vi "Inline Read.vi"(1 "RT Data in":T1 {"Device Channels"."Status"."BD Refs"."Data Reference" format="%.0x"; "Device Channels"."Command"."BD Refs"."Data Reference" format="%.0x"; "Local Chassis"."FPGA"."VS ref" format="%.0x"; "Local Chassis"."RSI Modules"."VS ref" format="%.0x"; "Local Chassis"."VS ref" format="%.0x"; "Device ref" format="%.0x"; "EtherCAT Masters"."DS402 Drive ECAT Slaves"."VS ref" format="%.0x"; "EtherCAT Masters"."REM IO ECAT Slaves"."VS ref" format="%.0x"; "EtherCAT Masters"."Generic EtherCAT Slaves"."VS ref" format="%.0x"; "EtherCAT Masters"."VS ref" format="%.0x"; "EtherCAT Masters"."EtherCAT Slaves"."FPGA"."VS ref" format="%.0x"; "EtherCAT Masters"."EtherCAT Slaves"."RSI Modules"."VS ref" format="%.0x"; "EtherCAT Masters"."EtherCAT Slaves"."VS ref" format="%.0x"}) -> (0 "RT Data out":T1 {"Device Channels"."Status"."BD Refs"."Data Reference" format="%.0x"; "Device Channels"."Command"."BD Refs"."Data Reference" format="%.0x"; "Local Chassis"."FPGA"."VS ref" format="%.0x"; "Local Chassis"."RSI Modules"."VS ref" format="%.0x"; "Local Chassis"."VS ref" format="%.0x"; "Device ref" format="%.0x"; "EtherCAT Masters"."DS402 Drive ECAT Slaves"."VS ref" format="%.0x"; "EtherCAT Masters"."REM IO ECAT Slaves"."VS ref" format="%.0x"; "EtherCAT Masters"."Generic EtherCAT Slaves"."VS ref" format="%.0x"; "EtherCAT Masters"."VS ref" format="%.0x"; "EtherCAT Masters"."EtherCAT Slaves"."FPGA"."VS ref" format="%.0x"; "EtherCAT Masters"."EtherCAT Slaves"."RSI Modules"."VS ref" format="%.0x"; "EtherCAT Masters"."EtherCAT Slaves"."VS ref" format="%.0x"})   [LabVIEW 2016, in "Scan Engine Custom Device.lvlib"]
uses:
  Scan Engine Custom Device.lvlib
  Type Defs/RT Data.ctl
  <vilib>/NI Veristand/Custom Device API/Custom Device Item Ref.ctl
  Type Defs/Device Channels.ctl
  Type Defs/Output Data.ctl
  <vilib>/NI Veristand/Custom Device API/Block Data Reference.ctl
  <vilib>/NI Veristand/Custom Device API/Data Reference.ctl
  Type Defs/Input Data.ctl
  Type Defs/Local Chassis Data.ctl
  Type Defs/RSI Module Data.ctl
  Type Defs/Open Module IOVs.ctl
  Modules.lvlibp/RSI Module/RSI Module.lvclass
  Modules.lvlibp/RSI Module/Module Models.ctl
  Modules.lvlibp/RSI Module/Channel Type.ctl
  Type Defs/Module Config Data.ctl
  Type Defs/Mixed IO.ctl
  Type Defs/FPGA Data.ctl
  Type Defs/UDV Data.ctl
  Type Defs/UDV Data Type.ctl
  Type Defs/FXP Config.ctl
  Type Defs/Mod Size Indexes.ctl
  Type Defs/EtherCAT Master Data.ctl
  Type Defs/EtherCAT Slave Data.ctl
  Type Defs/Generic ECAT Slave RT-Data-Array.ctl
  Type Defs/Generic ECAT Slave Data Cluster.ctl
  Type Defs/Generic ECAT Slave IOV Cluster.ctl
  Type Defs/REM IO ECAT Slave RT-Data-Array.ctl
  Type Defs/REM IO ECAT Slave Data Cluster.ctl
  Type Defs/REM IO ECAT Slave IOV Cluster.ctl
  Type Defs/DS402 Drive ECAT Slave RT-Data-Array.ctl
  Type Defs/DS402 Drive ECAT Slave Data Cluster.ctl
  Type Defs/DS402 Drive ECAT Slave IOV Cluster.ctl
  Type Defs/DS402 Drive ECAT Slave Action IOV Cluster.ctl
  Type Defs/Async Data.ctl
  Type Defs/Async Status.ctl
  Type Defs/Async State.ctl
  Type Defs/Async Command.ctl
  Type Defs/ECAT Reconfig Data.ctl
  Type Defs/ECAT Reconfig Status.ctl
  Type Defs/ECAT Reconfig State.ctl
  Type Defs/RW Case.ctl
  RW All Local.vi
  RW All ECAT.vi
  Check Command Channels.vi
  Read Async FIFOs.vi
  Update Status Channels.vi
  Module Reconfig/Check ECAT Reconfig.vi
  Write Async FIFOs.vi
  RW Local Chassis.vi
  RW Slave.vi
  RW Generic Slaves.vi
  RW Rem IO Slaves.vi
  RW DS402 Drive Slaves.vi
  <vilib>/NI Veristand/Custom Device API/NI VeriStand - Get Channel Values by Block Data Reference.vi
  <vilib>/NI Veristand/Custom Device API/NI VeriStand - Set Channel Values by Block Data Reference.vi
  RW UDVs.vi
  RW Mods.vi
  Read ECAT VARs.vi
  Write ECAT VARs.vi
  Read REM IO VARs.vi
  Write REM IO VARs.vi
  Read DS402 Drive VARs.vi
  Write DS402 Drive VARs.vi
  Read UDVs.vi
  Write UDVs.vi
  Read All Input Module Sizes.vi
  Read All Mixed Module Sizes.vi
  Write Module.vi
  Check Module Config.vi
  Scanned Read - UDV.vi
  Scanned Write - UDV.vi
  Read Input Modules at Indexes.vi
  Read Mixed Modules at Indexes.vi
  Scanned Write - Module.vi
  Read Input Module.vi
  Read Mixed Module.vi
  Scanned Read - Input Module.vi
  Scanned Read - Mixed Module.vi
  <vilib>/NI Veristand/Custom Device API/Global Data Refs.vi
  Module Reconfig/Set ECAT Reconfig Status.vi
  <vilib>/NI/syslog/Syslog Device Send.vi
  Launch Local Reconfig.vi
  DS402 StateMachine/Process DS402 SM.vi
  Async/Set Async Status.vi
  Launch ECAT Reconfig.vi
  Globals/Error Strings.vi
  Module Reconfig/Get ECAT Reconfig Status.vi
  Get Scan Mode.vi
  <vilib>/NI Veristand/Custom Device API/Custom Device API.lvlib
types:
  T1 = typedef "Scan Engine Custom Device.lvlib/RT Data.ctl" = cluster{"Device ref":T2, "Scan Period (uSec)":u32, "Device Channels":T3, "Local Chassis":T8[], "EtherCAT Masters":T20[], "Async":T32, "ECAT Reconfig":T33, "Device Error":errorcluster, "DeviceName":string, "PCLSync?":bool}
  T2 = typedef "Custom Device API.lvlib/Custom Device Item Ref.ctl" = u64
  T3 = typedef "Scan Engine Custom Device.lvlib/Device Channels.ctl" = cluster{"Status":T4, "Command":T7}
  T4 = typedef "Scan Engine Custom Device.lvlib/Output Data.ctl" = cluster{"BD Refs":T5[], "Length":i32, "FIFO Index":i32, "Data":dbl[]}
  T5 = typedef "Custom Device API.lvlib/Block Data Reference.ctl" = cluster{"Data Reference":T6, "Offset":u64, "Length":u64}
  T6 = typedef "Custom Device API.lvlib/Data Reference.ctl" = i32
  T7 = typedef "Scan Engine Custom Device.lvlib/Input Data.ctl" = cluster{"BD Refs":T5[], "Data":dbl[], "Length":i32, "FIFO Index":i32}
  T8 = typedef "Scan Engine Custom Device.lvlib/Local Chassis Data.ctl" = cluster{"VS ref":T2, "RSI Modules":T9[], "FPGA":T15[], "Input Mod Size Idxs":T19, "Output Modules":i32[], "MixedIO Mod Size Idxs":T19}
  T9 = typedef "Scan Engine Custom Device.lvlib/RSI Module Data.ctl" = cluster{"VS ref":T2, "IOV ref":refnum<k21>, "Open Mod refs":T10, "Module DVR":refnum<data-value>, "Slot":u32, "Model":T11, "Channel Type":T12, "EtherCAT?":bool, "CDInput Data":T7, "CDOutput Data":T4, "Module Config Data":T13, "Mixed IO":T14}
  T10 = typedef "Scan Engine Custom Device.lvlib/Open Module IOVs.ctl" = cluster{"Analog Read":refnum<k21>, "Digital Read":refnum<k21>, "Analog Write":refnum<k21>, "Digital Write":refnum<k21>}
  T11 = typedef "Modules.lvlibp/RSI Module.lvclass/Module Models.ctl" = enum16{"Empty", "NI 9201", "NI 9203", "NI 9205", "NI 9206", "NI 9207", "NI 9208", "NI 9211", "NI 9212", "NI 9213", "NI 9214", "NI 9215", "NI 9217", "NI 9219", "NI 9220", "NI 9221", "NI 9222", "NI 9223", "NI 9225", "NI 9227", "NI 9229", "NI 9233", "NI 9234", "NI 9235", "NI 9236", "NI 9237", "NI 9239", "NI 9242", "NI 9244", "NI 9263", "NI 9264", "NI 9265", "NI 9269", "NI 9375", "NI 9401", "NI 9402", "NI 9403", "NI 9411", "NI 9421", "NI 9422", "NI 9423", "NI 9425", "NI 9426", "NI 9435", "NI 9437", "NI 9472", "NI 9474", "NI 9475", "NI 9476", "NI 9477", "NI 9478", "NI 9481", "NI 9482", "NI 9485"}
  T12 = typedef "Modules.lvlibp/RSI Module.lvclass/Channel Type.ctl" = enum16{"Analog", "Digital"}
  T13 = typedef "Scan Engine Custom Device.lvlib/Module Config Data.ctl" = cluster{"Configurable?":bool, "Config Block Data Refs":T5[], "Config Data DVR":refnum<data-value>, "Previous Values":dbl[], "Local Reconfig VI Ref":refnum<vi>}
  T14 = typedef "Scan Engine Custom Device.lvlib/Mixed IO.ctl" = cluster{"Input Channel Indices":i32[], "Input Buffer":dbl[]}
  T15 = typedef "Scan Engine Custom Device.lvlib/FPGA Data.ctl" = cluster{"VS ref":T2, "IOV ref":refnum<k21>, "FPGA Target":enum16{"Local", "EtherCAT"}, "Product Code":u32, "Bitfile Signature":string, "Bitfile Path (RT)":path, "FPGA Session":u32, "Input Data":T7, "Output Data":T4, "UDVs":cluster{"From FPGA":T16[], "To FPGA":T16[]}}
  T16 = typedef "Scan Engine Custom Device.lvlib/UDV Data.ctl" = cluster{"VS ref":T2, "IOV Ref":refnum<k21>, "Name":string, "UDV Data Type":T17, "Supported Type?":bool, "FXP Config":T18, "FXP VI Ref":refnum<vi>}
  T17 = typedef "Scan Engine Custom Device.lvlib/UDV Data Type.ctl" = enum16{"Boolean", "Fixed Point", "Int8", "Int16", "Int32", "Int64", "U32 Bit Field", "UInt8", "UInt16", "UInt32", "UInt64", "Other"}
  T18 = typedef "Scan Engine Custom Device.lvlib/FXP Config.ctl" = cluster{"signed":bool, "size":u32, "integersize":i32}
  T19 = typedef "Scan Engine Custom Device.lvlib/Mod Size Indexes.ctl" = cluster{"4":i32[], "8":i32[], "16":i32[], "32":i32[], "other":i32[]}
  T20 = typedef "Scan Engine Custom Device.lvlib/EtherCAT Master Data.ctl" = cluster{"VS ref":T2, "IOV ref":refnum<k21>, "Master ID":u32, "Cyclic Data Bandwidth":u32, "EtherCAT Slaves":T21[], "Generic EtherCAT Slaves":T22, "REM IO ECAT Slaves":T25, "DS402 Drive ECAT Slaves":T28}
  T21 = typedef "Scan Engine Custom Device.lvlib/EtherCAT Slave Data.ctl" = cluster{"VS ref":T2, "IOV ref":refnum<k21>, "Position Address":u16, "RSI Modules":T9[], "FPGA":T15[], "Input Mod Size Idxs":T19, "Output Modules":i32[], "MixedIO Mod Size Idxs":T19}
  T22 = typedef "Scan Engine Custom Device.lvlib/Generic ECAT Slave RT-Data-Array.ctl" = T23[]
  T23 = typedef "Scan Engine Custom Device.lvlib/Generic ECAT Slave Data Cluster.ctl" = cluster{"VS ref":T2, "IOV ref":refnum<k21>, "Position Address":u16, "I/O Imput Vars ":T24[], "I/O Output Vars":T24[], "I/O Input Data":T7, "I/O Output Data":T4}
  T24 = typedef "Scan Engine Custom Device.lvlib/Generic ECAT Slave IOV Cluster.ctl" = cluster{"VS ref":T2, "IOV Ref":refnum<k21>, "Name":string, "UDV Data Type":T17}
  T25 = typedef "Scan Engine Custom Device.lvlib/REM IO ECAT Slave RT-Data-Array.ctl" = T26[]
  T26 = typedef "Scan Engine Custom Device.lvlib/REM IO ECAT Slave Data Cluster.ctl" = cluster{"VS ref":T2, "IOV ref":refnum<k21>, "Position Address":u16, "I/O Imput Vars ":T27[], "I/O Output Vars":T27[], "I/O Input Data":T7, "I/O Output Data":T4}
  T27 = typedef "Scan Engine Custom Device.lvlib/REM IO ECAT Slave IOV Cluster.ctl" = cluster{"VS ref":T2, "IOV Ref":refnum<k21>, "Name":string, "UDV Data Type":T17, "Scaling Factor":dbl}
  T28 = typedef "DS402 Drive ECAT Slave RT-Data-Array.ctl" = T29[]
  T29 = typedef "Scan Engine Custom Device.lvlib/DS402 Drive ECAT Slave Data Cluster.ctl" = cluster{"VS ref":T2, "IOV ref":refnum<k21>, "Position Address":u16, "I/O Input Vars ":T30[], "I/O Output Vars":T30[], "I/O Input Data":T7, "I/O Output Data":T4, "DS402 IOV":T31}
  T30 = typedef "Scan Engine Custom Device.lvlib/DS402 Drive ECAT Slave IOV Cluster.ctl" = cluster{"VS ref":T2, "IOV Ref":refnum<k21>, "Name":string, "UDV Data Type":T17, "Scaling Factor":dbl, "IOV":bool, "VS data Index":i32}
  T31 = typedef "Scan Engine Custom Device.lvlib/DS402 Drive ECAT Slave Action IOV Cluster.ctl" = cluster{"Control Word":refnum<k21>, "Status Word":refnum<k21>}
  T32 = typedef "Scan Engine Custom Device.lvlib/Async Data.ctl" = cluster{"Status":refnum<queue>, "Command":refnum<queue>, "Input FIFO":refnum<k33>, "Input FIFO buffer":dbl[], "Output FIFO":refnum<k33>, "Output FIFO buffer":dbl[], "Async VI Ref":refnum<vi>}
  T33 = typedef "Scan Engine Custom Device.lvlib/ECAT Reconfig Data.ctl" = cluster{"Reconfig Module Found":bool, "VI Ref":refnum<vi>, "Status":refnum<queue>}
  T34 = typedef "Scan Engine Custom Device.lvlib/RW Case.ctl" = enum16{"Inline read", "Inline write", "Async - Inline loop read", "Async - Inline loop write", "Async loop (read/write)"}
  T35 = typedef "Scan Engine Custom Device.lvlib/Async State.ctl" = enum16{"Not running", "Waiting on start cmd", "Running", "Paused", "Stopped"}
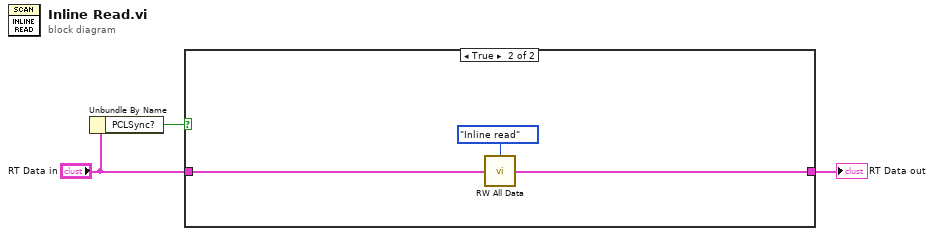
[diagram p0: block diagram]
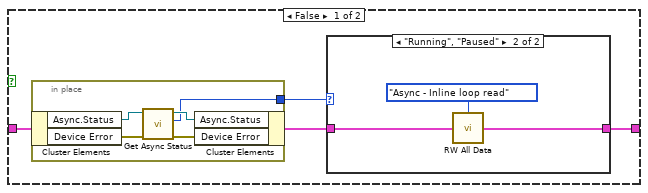
[diagram p2: hidden frame]
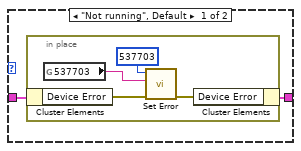
[diagram p3: hidden frame]
diagram:
  n1 = Unbundle By Name("RT Data in") -> ("PCLSync?"=w1:bool)
  n2 = case shown="True" w1 {
    tunnel: "RT Data in" -> [w7 w23]
    tunnel: [w4 w22] -> w3
    frame False {
      n3 = in-place {
        in-place-border: [w17] -> w6
        n4 = in-place-cluster #1(w7) -> ("Async.Status"=w21:refnum<queue>, "Device Error"=w20:errorcluster)
        n5 = call "Get Async Status.vi"("error in (no error)"=w20, "Status in"=w21) -> ("error out"=w18:errorcluster, "State"=w17:T35, "Status out"=w19:refnum<queue>)  [unwired: 7 in]
        n6 = in-place-cluster #1("Async.Status"=w19, "Device Error"=w18) -> (w5:T1)
      }
      n7 = case shown="\"Running\", \"Paused\"" w6 {
        tunnel: w5 -> [w9 w16]
        tunnel: [w8 w14] -> w4
        frame "Not running", Default {
          n8 = in-place {
            n9 = in-place-cluster #2(w9) -> ("Device Error"=w13:errorcluster)
            n10 = global read "Error Strings.vi" "537703"() -> (w10:string)
            n11 = call "Set Error.vi"("error in (no error)"=w13, "Message"=w10, "Code"=537703 ("error code (0)")) -> ("error out"=w12:errorcluster)  [unwired: 8 in]
            n12 = in-place-cluster #2("Device Error"=w12) -> (w8:T1)
          }
        }
        frame "Running", "Paused" {
          n13 = call "RW All Data.vi"("R/W Case"=RW_Case."Async - Inline loop read", "RT Data in"=w16) -> ("RT Data out"=w14:T1)  [unwired: 13 in]
        }
      }
    }
    frame True {
      n14 = call "RW All Data.vi"("R/W Case"=RW_Case."Inline read", "RT Data in"=w23) -> ("RT Data out"=w22:T1)  [unwired: 13 in]
    }
  }
  "RT Data out" <- w3
